vi "check pointer.vi"(11 "pointer in":u64) -> (2 "ok":bool, 3 "pointer out":u64)   [LabVIEW 2020, in "libpcaplv.lvlib"]
uses:
  libpcaplv.lvlib
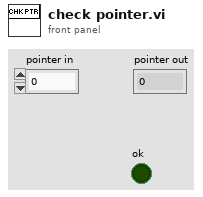
[diagram p1: front panel]
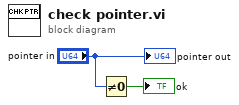
[diagram p0: block diagram]
diagram:
  n1 = Not Equal To 0?(x="pointer in") -> (x != 0?=→"ok":bool)
  "pointer out" <- "pointer in"
